vi "Destroy.vi"(8 "error in (no error)":errorcluster, 11 "DataSocketMessenger in":refnum<class "DataSocketMessenger.lvclass">) -> (0 "error out":errorcluster)   [LabVIEW 2011, in "Messenging.lvlib" / "DataSocketMessenger.lvclass"]
uses:
  DataSocketMessenger.lvclass
  DataSocketMessenger.lvclass/DataSocketMessenger.ctl
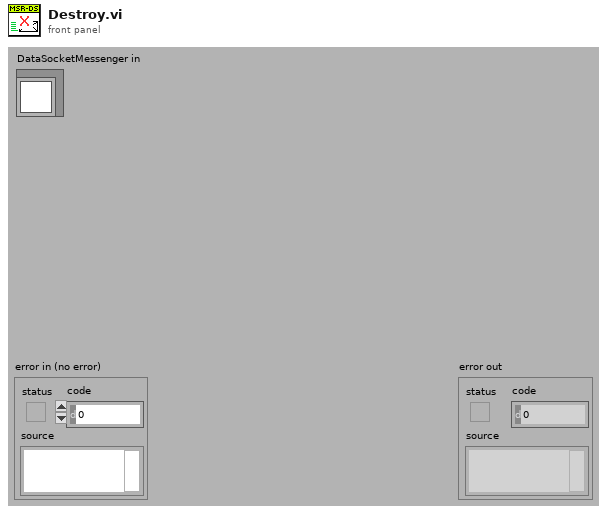
[diagram p1: front panel]
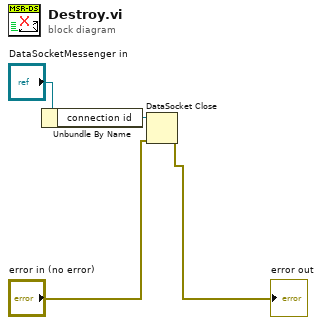
[diagram p0: block diagram]
diagram:
  n1 = Unbundle By Name("DataSocketMessenger in") -> ("connection id"=w3:refnum<k13>)
  n2 = DataSocket Close(8:"error in (no error)", 11:w3) -> (0:→"error out":errorcluster)  [unwired: 2 out]
